vi "Actor Core.vi"(8 "error in":errorcluster, 11 "Nested in":refnum<class "User Interface.lvclass">) -> (0 "error out":errorcluster, 3 "Actor out":refnum<class "Actor.lvclass">)   [LabVIEW 2020, in "User Interface.lvlib" / "User Interface.lvclass"]
doc: "(<B>Filename</B>: Actor Framework.lvlib:Actor.lvclass:Actor Core.vi)\n\nReceives messages to the actor, reacts to them, and initiates any error handling that may shut the actor down.\n\nDescendant classes may override this VI to append parallel tasks for the actor to complete while it handles messages. Overrides use the Call Parent Method node."
uses:
  User Interface.lvclass
  C:/Program Files (x86)/National Instruments/LabVIEW 2020/vi.lib/ActorFramework/Actor/Actor.lvclass
  <vilib>/ActorFramework/Actor/Actor.lvclass
  <vilib>/ActorFramework/Actor/Actor.lvclass/Actor.ctl
  <vilib>/ActorFramework/Message Enqueuer/Message Enqueuer.lvclass/Message Enqueuer.ctl
  User Interface.lvclass/User Interface.ctl
  Businness Logic/Businness Logic Messages/Start_Stop Aq Msg/Start_Stop Aq Msg.lvclass/Start_Stop Aq Msg.ctl
  <vilib>/ActorFramework/Message Enqueuer/Init from Existing Queue.vi
  <vilib>/ActorFramework/Message Enqueuer/Enqueue.vi
  <vilib>/ActorFramework/Stop Msg/Stop Msg.lvclass
  C:/Program Files (x86)/National Instruments/LabVIEW 2020/vi.lib/ActorFramework/Message/Message.lvclass
  Businness Logic/Businness Logic Messages/Start_Stop Aq Msg/Start_Stop Aq Msg.lvclass
  <vilib>/ActorFramework/Message Priority Queue/Priority Enqueue.vi
  <vilib>/ActorFramework/Message Enqueuer/Message Enqueuer.lvclass
  D:/Storage/Source Code/Clase AF/ClaseAF/08 Acquisition AF/User Interface/User Interface.lvclass
panel:
  out "Data":dbl[](graph)
  in  "Stop":bool
  in  "Start":bool
  out "Status":string
  in  "Exit":bool
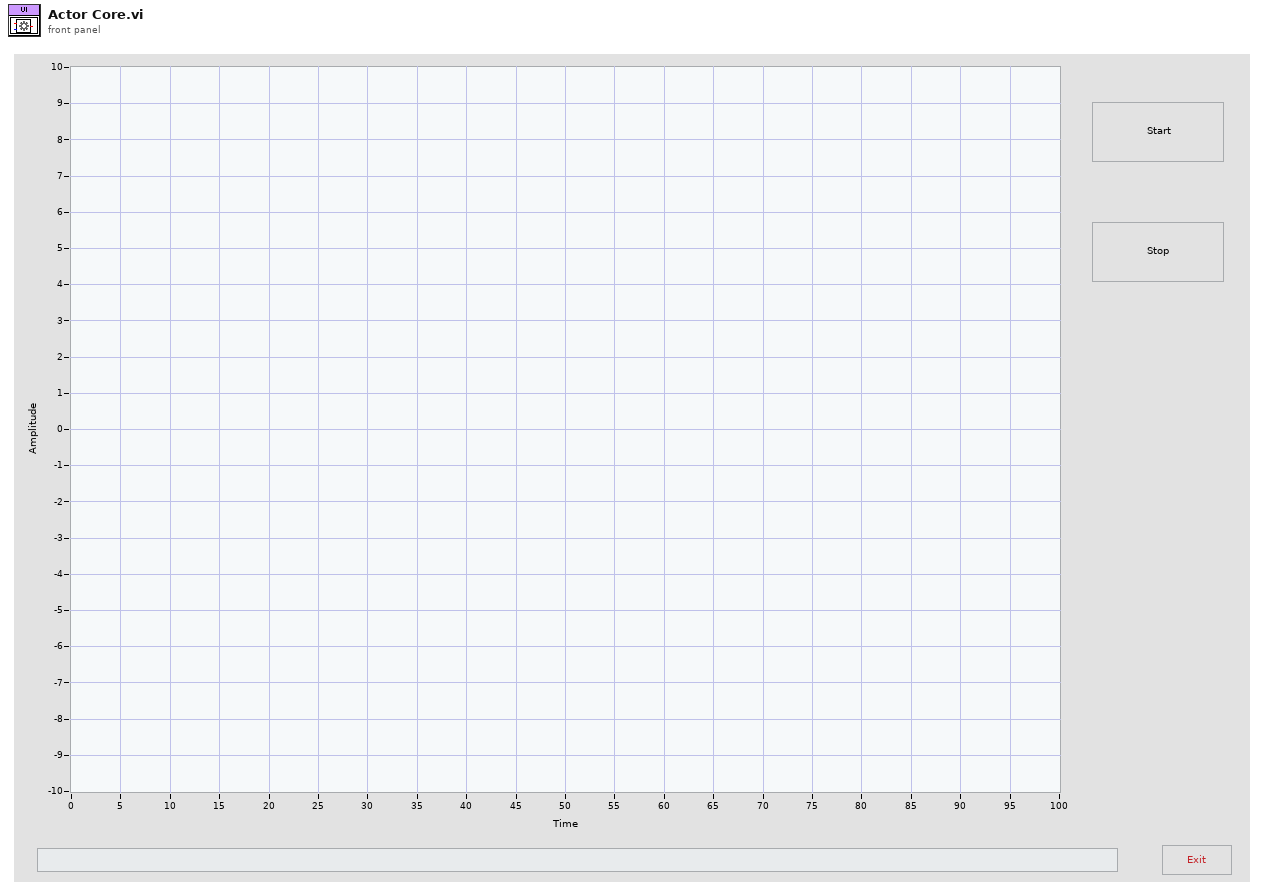
[diagram p1: front panel]
types:
  T1 = cluster{"Stop":refnum<user-event>, "Data":refnum<user-event>, "Status":refnum<user-event>}
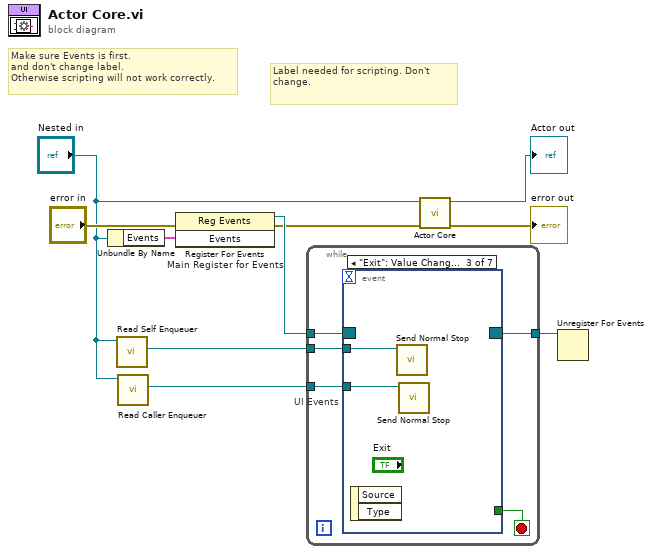
[diagram p0: block diagram]
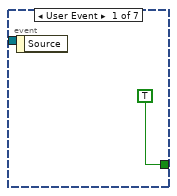
[diagram p2: hidden frame]
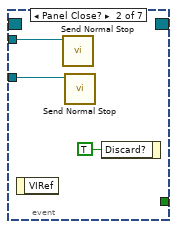
[diagram p3: hidden frame]
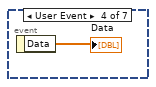
[diagram p4: hidden frame]
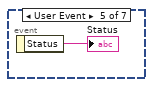
[diagram p5: hidden frame]
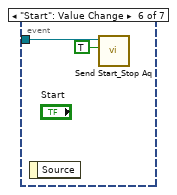
[diagram p6: hidden frame]
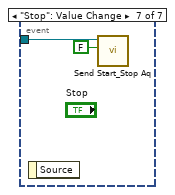
[diagram p7: hidden frame]
diagram:
  # "Label needed for scripting. Don't change."
  # "Make sure Events is first.\nand don't change label.\nOtherwise scripting will not work correctly."
  n1 = Unbundle By Name("Nested in") -> ("Events"=w7:T1)
  n2 = call <vilib>:"Read Self Enqueuer.vi"("Actor"="Nested in") -> ("Self Enqueuer"=w5:refnum<class "Message Enqueuer.lvclass">)  [unwired: 10 in]
  n3 = call <vilib>:"Read Caller Enqueuer.vi"("Actor"="Nested in") -> ("Caller Enqueuer"=w1:refnum<class "Message Enqueuer.lvclass">)  [unwired: 10 in]
  n4 = register-events "Main Register for Events"(error in="error in", w7) -> (reference out=w8:refnum<event-registration>, error out=w3:errorcluster)  [unwired: 1 in]
  n5 = while {
    tunnel: w8 -> [w15]
    tunnel: [w13] -> w6
    tunnel: w5 -> [w12]
    tunnel: w1 -> [w11]
    stop <- w14 stop-if-true
    n6 = event "UI Events" shown="[2] \"Exit\": Value Change" {
      selector: w15 -> [_ _ _ _ _ _ _]
      dyn-events: [_ _ _ _ _ _ _] -> w13
      timeout: _ -> [_ _ _ _ _ _ _]
      tunnel: [TRUE _ _ _ _ _ _] -> w14
      tunnel: w12 -> [_ w18 w21 _ _ _ _]
      tunnel: w11 -> [_ w17 w20 _ _ w25 w27]
      event User Event {
        n7 = event-data() -> ()  [unwired: 1 in, 1 out]
      }
      event Panel Close? {
        n8 = event-data() -> ()  [unwired: 1 in, 1 out]
        n9 = call <vilib>:"Send Normal Stop.vi"("Message Enqueuer"=w18) -> ()  [unwired: 10 in, 1 out]
        n10 = call <vilib>:"Send Normal Stop.vi"("Message Enqueuer"=w17) -> ()  [unwired: 10 in, 1 out]
        n11 = event-data("Discard?"=TRUE) -> ()  [unwired: 1 in, 1 out]
      }
      event "Exit": Value Change {
        n12 = event-data() -> ()  [unwired: 1 in, 2 out]
        n13 = call <vilib>:"Send Normal Stop.vi"("Message Enqueuer"=w21) -> ()  [unwired: 10 in, 1 out]
        n14 = call <vilib>:"Send Normal Stop.vi"("Message Enqueuer"=w20) -> ()  [unwired: 10 in, 1 out]
      }
      event User Event {
        n15 = event-data() -> ("Data"=→"Data":dbl[])  [unwired: 1 in]
      }
      event User Event {
        n16 = event-data() -> ("Status"=→"Status":string)  [unwired: 1 in]
      }
      event "Start": Value Change {
        n17 = event-data() -> ()  [unwired: 1 in, 1 out]
        n18 = call "Send Start_Stop Aq.vi"("Start/Stop AQ"=TRUE, "Message Enqueuer"=w25) -> ()  [unwired: 8 in, 2 out]
      }
      event "Stop": Value Change {
        n19 = event-data() -> ()  [unwired: 1 in, 1 out]
        n20 = call "Send Start_Stop Aq.vi"("Start/Stop AQ"=FALSE, "Message Enqueuer"=w27) -> ()  [unwired: 8 in, 2 out]
      }
    }
  }
  n21 = call-parent "Actor Core.vi"("error in"=w3, "Actor in"="Nested in") -> ("error out"=→"error out":errorcluster, "Actor out"=→"Actor out":refnum<class "Actor.lvclass">)  [unwired: 8 in]
  n22 = Unregister For Events(event registration refnum=w6) -> ()  [unwired: 1 in, 1 out]
